vi "Update Subpanel Refs.vi"(8 "error in":errorcluster, 9 "subpanel UIDs":i32[](array[numeric]), 10 "subpanel refnums":refnum<vi>[](array[refnum]), 11 "VI info in":T1) -> (0 "error out":errorcluster, 3 "VI info out":T1)   [LabVIEW 2010, in "NI_SE_Config Front Panel Layout.lvlib"]
uses:
  NI_SE_Config Front Panel Layout.lvlib
  VI Info.ctl
  VI Panel Layout/VI Panel Layout.lvclass
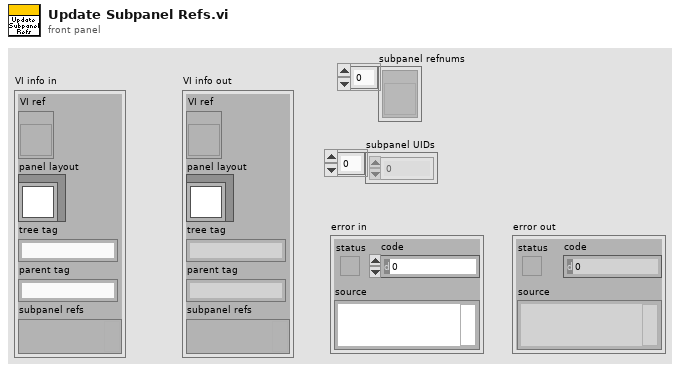
[diagram p1: front panel]
types:
  T1 = typedef "NI_SE_Config Front Panel Layout.lvlib/VI Info.ctl" = cluster{"VI ref":refnum<vi>, "panel layout":refnum<class "VI Panel Layout.lvclass">, "tree tag":string, "parent tag":string, "subpanel refs":variant}
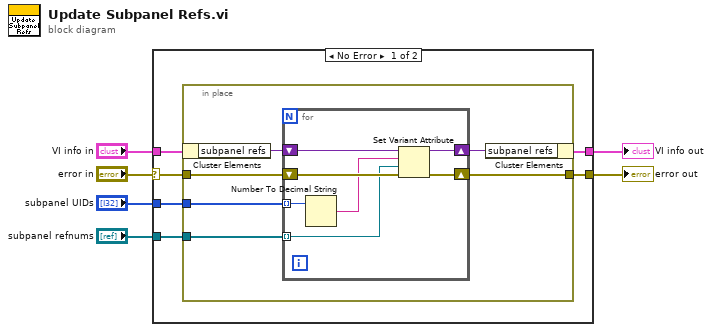
[diagram p0: block diagram]
diagram:
  n1 = case shown="No Error" "error in" {
    selector: "error in" -> [w10 w27]
    tunnel: "VI info in" -> [w12 w26]
    tunnel: [w9 w27] -> w4
    tunnel: [w11 w26] -> w3
    tunnel: "subpanel UIDs" -> [w8 _]
    tunnel: "subpanel refnums" -> [w7 _]
    frame No Error {
      n2 = in-place {
        in-place-border: w10 -> [w16]
        in-place-border: [w15] -> w9
        in-place-border: w8 -> [w14]
        in-place-border: w7 -> [w13]
        n3 = in-place-cluster #1(w12) -> ("subpanel refs"=w18:variant)
        n4 = for {
          shift-right: [w25] -> w17
          shift-left: w18 -> [w19]
          shift-right: [w23] -> w15
          shift-left: w16 -> [w24]
          tunnel: w14 -> [w22] mode=indexing
          tunnel: w13 -> [w20] mode=indexing
          n5 = Number To Decimal String(number=w22) -> (decimal integer string=w21:string)  [unwired: 1 in]
          n6 = Set Variant Attribute(Variant=w19, name=w21, value=w20, error in=w24) -> (Variant out=w25:variant, error out=w23:errorcluster)  [unwired: 1 out]
        }
        n7 = in-place-cluster #1("subpanel refs"=w17) -> (w11:T1)
      }
    }
    frame Error {
    }
  }
  "VI info out" <- w3
  "error out" <- w4
